vi "Get Max Sub-Index.vi"(8 "Error In":errorcluster, 11 "reference in":refnum<class "OD Entry.lvclass">) -> (0 "Error Out":errorcluster, 2 "Max Sub-Index":u8, 3 "reference out":refnum<class "OD Entry.lvclass">)   [LabVIEW 2024, in "EDS.lvlib" / "OD Entry.lvclass"]
doc: "Return max indicated subindex, or null if not array or record"
uses:
  OD Entry.lvclass
  OD Entry.lvclass/OD Entry.ctl
  Object Type.ctl
  EDS.lvlib
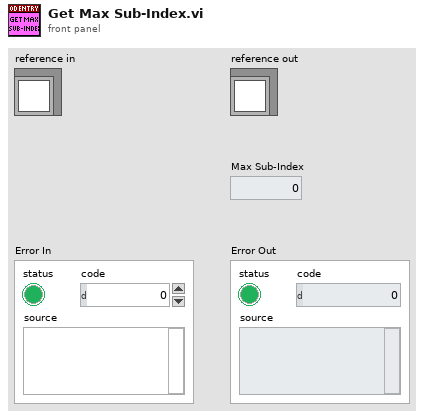
[diagram p1: front panel]
types:
  T1 = typedef "EDS.lvlib/Object Type.ctl" = i16
  T2 = typedef "EDS.lvlib/OD Entry.lvclass/ObjectAttributes.ctl" = cluster{"Index":u16, "ParameterName":string, "Denotation":string, "ObjectType":T1, "DataType":T3, "AccessType":T4, "DefaultValue":string, "LowLimit":string, "HighLimit":string, "ObjFlags":u32, "CompactSubObj":u8, "PDOMapping":bool, "Count":u8, "ObjExtend":u8, "PDOtype":T5, "Label":string, "Description":string, "Sub-Entries":map{u16, refnum<class "OD Sub-Entry.lvclass">}}
  T3 = typedef "EDS.lvlib/Data Type.ctl" = enum16{"UNKNOWN", "BOOLEAN", "INTEGER8", "INTEGER16", "INTEGER32", "UNSIGNED8", "UNSIGNED16", "UNSIGNED32", "REAL32", "VISIBLE_STRING", "OCTET_STRING", "UNICODE_STRING", "TIME_OF_DAY", "TIME_DIFFERENCE", "RESERVED1", "DOMAIN", "INTEGER24", "REAL64", "INTEGER40", "INTEGER48", "INTEGER56", "INTEGER64", "UNSIGNED24", "RESERVED2", "UNSIGNED40", "UNSIGNED48", "UNSIGNED56", "UNSIGNED64", "RESERVED3", "RESERVED4", "RESERVED5", "RESERVED6", "PDO_COMMUNICATION_PARAMETER", "PDO_MAPPING", "SDO_PARAMETER", "IDENTITY", "RESERVED7"}
  T4 = typedef "EDS.lvlib/Access Type.ctl" = enum16{"rw", "ro", "wo", "rwr", "rww", "const", "UNKNOWN"}
  T5 = typedef "EDS.lvlib/PDO Mapping Type.ctl" = enum16{"NO", "OPTIONAL", "RPDO", "TPDO", "DEFAULT"}
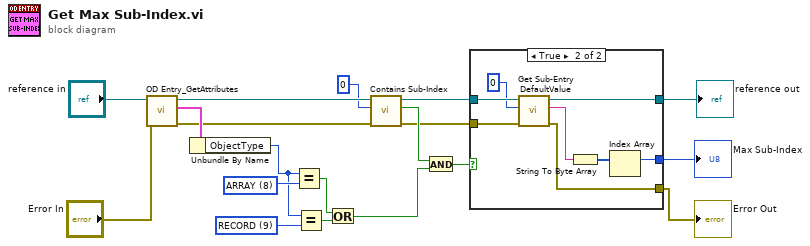
[diagram p0: block diagram]
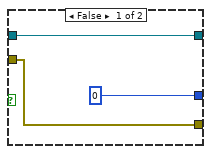
[diagram p2: hidden frame]
diagram:
  w12 = T1 9 items=["UNKNOWN"=-1, "NULL"=0, "DOMAIN"=2, "DEFTYPE"=5, "DEFSTRUCT"=6, "VAR"=7, "ARRAY"=8, "RECORD"=9] ("y")
  w15 = T1 8 items=["UNKNOWN"=-1, "NULL"=0, "DOMAIN"=2, "DEFTYPE"=5, "DEFSTRUCT"=6, "VAR"=7, "ARRAY"=8, "RECORD"=9] ("y")
  n1 = call "OD Entry_GetAttributes.vi"("Error In"="Error In", "reference in"="reference in") -> ("Error Out"=w9:errorcluster, "Data"=w16:T2, "reference out"=w17:refnum<class "OD Entry.lvclass">)  [unwired: 6 in, 1 out]
  n2 = Unbundle By Name(w16) -> ("ObjectType"=w13:T1)
  n3 = Equal?(x=w13, y=w15) -> (x = y?=w14:bool)
  n4 = Equal?(x=w13, y=w12) -> (x = y?=w8:bool)
  n5 = Or(x=w14, y=w8) -> (x .or. y?=w6:bool)
  n6 = call "Contains Sub-Index.vi"("Error In"=w9, "Sub-Index"=u16 0, "reference in"=w17) -> ("Error Out"=w2:errorcluster, "Contains?"=w7:bool, "reference out"=w11:refnum<class "OD Entry.lvclass">)  [unwired: 6 in]
  n7 = And(x=w7, y=w6) -> (x .and. y?=w4:bool)
  n8 = case shown="True" w4 {
    tunnel: w11 -> [w22 w30]
    tunnel: [w22 w29] -> w5
    tunnel: [u8 0 w25] -> w3
    tunnel: w2 -> [w20 w24]
    tunnel: [w20 w23] -> w1
    frame False {
    }
    frame True {
      n9 = call "Get Sub-Entry DefaultValue.vi"("Error In"=w24, "Sub-Index"=u16 0, "reference in"=w30) -> ("Error Out"=w23:errorcluster, "DefaultValue"=w27:string, "reference out"=w29:refnum<class "OD Entry.lvclass">)  [unwired: 5 in, 1 out]
      n10 = String To Byte Array(string=w27) -> (unsigned byte array=w26:u8[])
      n11 = Index Array(array=w26) -> (element=w25:u8)  [unwired: 1 in]
    }
  }
  "Error Out" <- w1
  "reference out" <- w5
  "Max Sub-Index" <- w3
